vi "Semaphore Timed Wait (relative nanoseconds).vi"(8 "error in (no error)":errorcluster, 10 "relative timeout (nanoseconds)":i64, 11 "Semaphore in":T1) -> (0 "error out":errorcluster, 2 "timed out?":bool, 3 "Semaphore out":T1)   [LabVIEW 2013, in "POSIX Threads.lvlib" / "Semaphore.lvclass"]
doc: "Calls sem_timedwait() on the semaphore object encapsulated by Semaphore.\n\nThis VI attempts to decrement the value of the semaphore by 1 within a timeout period. If the semaphore can be decremented within the timeout period, this VI returns indicating it was successful. Otherwise, this VI returns indicating the semaphore was never set.\n\nRefer to online POSIX documentation for more information."
uses:
  Semaphore.lvclass
  Controls/reference.ctl
  <vilib>/NI/NI Linux RT Utilities/Controls/Public/C Enums/clockid_t.ctl
  POSIX Thread Object/POSIX Thread Object.lvclass/POSIX Thread Object.ctl
  POSIX Thread Object/Private VIs/libpthread path.vi
  <vilib>/NI/NI Linux RT Utilities/VIs/Public/Convert Types/convert timespec 64 to timespec 32.vi
  <vilib>/NI/NI Linux RT Utilities/VIs/Public/Time/Increment Time (timespec).vi
  <vilib>/NI/NI Linux RT Utilities/VIs/Public/Time/Get Clock Time (timespec).vi
  POSIX Thread Object/Private VIs/get pthread error.vi
  <vilib>/NI/NI Linux RT Errno/VIs/Public/Get Errno Value for Calling Thread.vi
  POSIX Thread Object/POSIX Thread Object.lvclass
  <vilib>/NI/NI Linux RT Utilities/Linux RT Utilities.lvlib
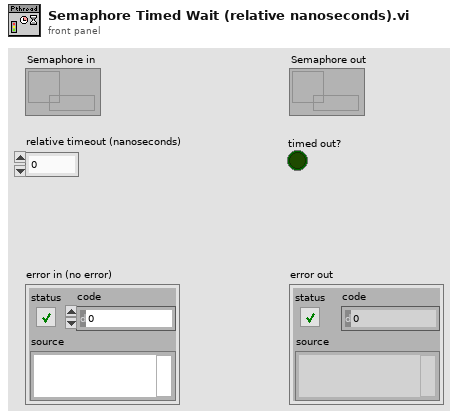
[diagram p1: front panel]
types:
  T1 = typedef "POSIX Threads.lvlib/Semaphore.lvclass/reference.ctl" = refnum<data-value>
  T2 = typedef "Linux RT Utilities.lvlib/clockid_t.ctl" = enum16{"Realtime", "Monotonic"}
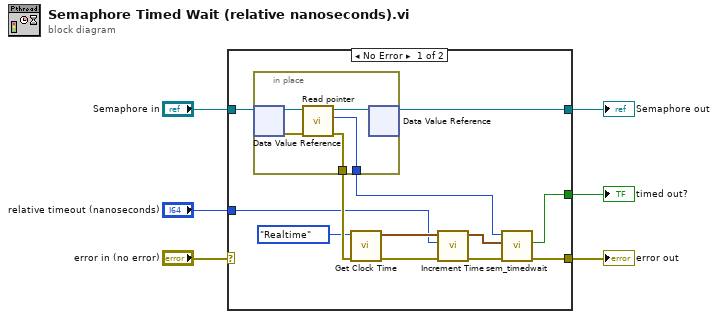
[diagram p0: block diagram]
diagram:
  n1 = case shown="No Error" "error in (no error)" {
    selector: "error in (no error)" -> [_ w24]
    tunnel: "Semaphore in" -> [w18 w25]
    tunnel: [w17 w25] -> w3
    tunnel: [w16 w24] -> w4
    tunnel: "relative timeout (nanoseconds)" -> [w7 _]
    tunnel: [w15 _] -> w1
    frame No Error {
      n2 = in-place {
        in-place-border: [w20] -> w13
        in-place-border: [w19] -> w14
        n3 = in-place-dvr #1(w18) -> (w23:refnum<class "Semaphore.lvclass">, w22:errorcluster)
        n4 = call "Read pointer.vi"("error in (no error)"=w22, "POSIX Thread Object in"=w23) -> ("error out"=w20:errorcluster, "pointer"=w19:u64, "POSIX Thread Object out"=w21:refnum<class "Semaphore.lvclass">)  [unwired: 7 in]
        n5 = in-place-dvr #1(w21) -> (w17:T1)  [unwired: 1 out]
      }
      n6 = call-poly <vilib>:"Get Clock Time.vi"("error in (no error)"=w13, "clock id (realtime)"=clockid_t."Realtime" ("clock id (monotonic)")) -> ("error out"=w11:errorcluster, "timespec"=w10:cluster{"sec":u64, "nsec":u64})  [unwired: 8 in]
      n7 = call-poly <vilib>:"Increment Time.vi"("error in (no error)"=w11, "nanoseconds to add"=w7, "timespec in"=w10) -> ("error out"=w8:errorcluster, "timespec out"=w9:cluster{"sec":u64, "nsec":u64})  [unwired: 7 in]
      n8 = call "sem_timedwait.vi"("error in (no error)"=w8, "absolute timeout"=w9, "sempahore ptr in"=w14) -> ("error out"=w16:errorcluster, "timed out?"=w15:bool)  [unwired: 6 in, 1 out]
    }
    frame Error {
    }
  }
  "error out" <- w4
  "Semaphore out" <- w3
  "timed out?" <- w1
